vi "Sweep VWL RESET.vi"(6 "Other Fixed Voltage (V)":dbl, 8 "error in (no error)":errorcluster, 10 "Pulse Width (us)":dbl, 11 "Sweep outfile":path) -> (0 "error out":errorcluster, 1 "final current (A)":dbl, 2 "final resistance (ohm)":dbl, 3 "final voltage (V)":dbl)   [LabVIEW 2019]
uses:
  Globals.vi
  <vilib>/Utility/file.llb/Write Delimited Spreadsheet (DBL).vi
panel:
  out "initial resistance (ohm)":dbl format="%#_6p"
  out "VSL (V)":dbl
  out "VBL (V)":dbl
  out "VWL (V)":dbl
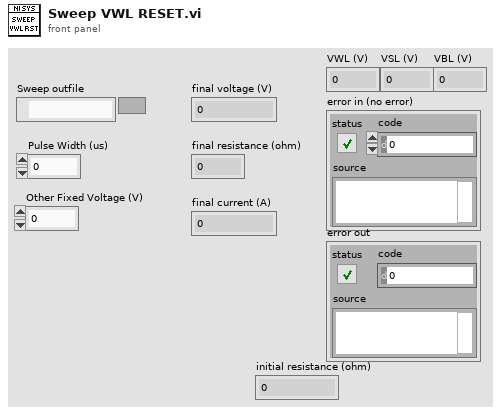
[diagram p1: front panel]
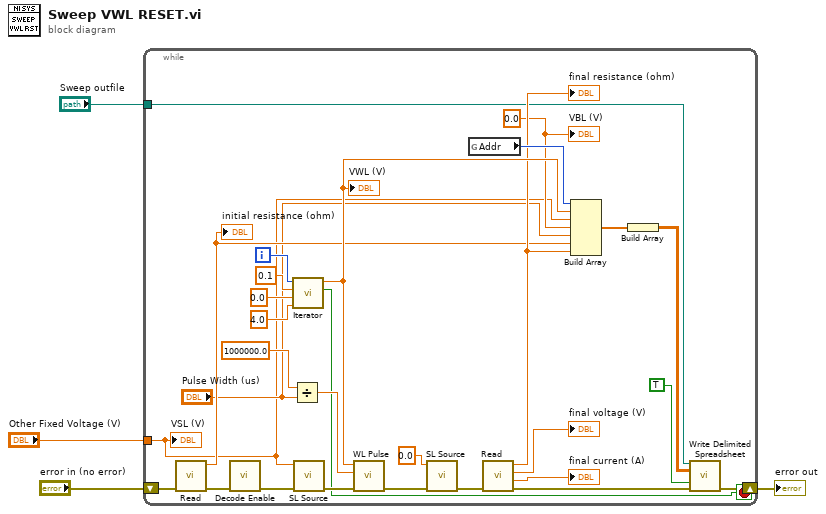
[diagram p0: block diagram]
diagram:
  n1 = while {
    tunnel: "Other Fixed Voltage (V)" -> [w6]
    shift-right: [w9] -> w1
    shift-left: "error in (no error)" -> [w23]
    tunnel: "Sweep outfile" -> [w13]
    i -> [w30]
    stop <- w16 stop-if-true
    w7 = 0.0 ("VSL (V)")
    n2 = call "Read.vi"("error in (no error)"=w23) -> ("error out"=w22:errorcluster, "resistance (ohm)"=w15:dbl)  [unwired: 7 in, 2 out]
    "initial resistance (ohm)" <- w15
    n3 = call "Decode Enable.vi"("error in (no error)"=w22) -> ("error out"=w29:errorcluster)  [unwired: 10 in]
    n4 = Divide(x=1000000.0 ("Sample Rate"), y="Pulse Width (us)") -> (x/y=w25:dbl)
    n5 = call "Iterator.vi"("Final Value"=4.0, "Initial Value"=0.0, "Step"=0.1, "i"=w30) -> ("End Loop"=w16:bool, "Current Value"=w20:dbl)  [unwired: 6 in]
    "VWL (V)" <- w20
    n6 = call "SL Source.vi"("error in (no error)"=w29, "voltage level (V)"=w6) -> ("error out"=w27:errorcluster)  [unwired: 9 in]
    n7 = call "WL Pulse.vi"("error in (no error)"=w27, "Sample Rate"=w25, "VWL (V)"=w20) -> ("error out"=w28:errorcluster)  [unwired: 8 in]
    n8 = call "SL Source.vi"("error in (no error)"=w28, "voltage level (V)"=0.0) -> ("error out"=w26:errorcluster)  [unwired: 9 in]
    n9 = global read "Globals.vi" "Addr"() -> (w21:u16)
    n10 = call "Read.vi"("error in (no error)"=w26) -> ("error out"=w12:errorcluster, "current (A)"=→"final current (A)":dbl, "read voltage (V)"=→"final voltage (V)":dbl, "resistance (ohm)"=w17:dbl)  [unwired: 7 in]
    "final resistance (ohm)" <- w17
    n11 = Build Array(w21, w20, w6, w7, "Pulse Width (us)", w15, w17) -> (w11:dbl[])
    n12 = Build Array(w11) -> (w10:dbl[][])
    n13 = call-poly <vilib>:"Write Delimited Spreadsheet.vi"("file path (dialog if empty)"=w13, "2D data"=w10, "append to file? (new file:F)"=TRUE, "error in (no error)"=w12) -> ("error out"=w9:errorcluster)  [unwired: 10 in, 1 out]
    "VSL (V)" <- w6
    "VBL (V)" <- w7
  }
  "error out" <- w1
